vi "Convert Event Level.vi"(4 "Event Level":T2=enum."Info") -> (7 "Enumeration":T1)   [LabVIEW 2020, in "Volatus.lvlib" / "Event Reporter Module.lvclass"]
uses:
  Event Reporter Module.lvclass
  Event Reporter Module.lvclass/Event Reporter Module.ctl
  messages/EventLevel/Enumeration.ctl
  messages/EventLevel/EventLevel.lvlib
  Event Level.ctl
  Volatus.lvlib
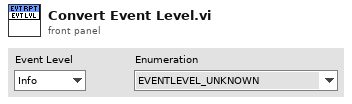
[diagram p1: front panel]
types:
  T1 = typedef "EventLevel.lvlib/Enumeration.ctl" = enum16{"EVENTLEVEL_UNKNOWN", "EVENTLEVEL_DEBUG", "EVENTLEVEL_INFO", "EVENTLEVEL_WARNING", "EVENTLEVEL_ERROR"}
  T2 = typedef "Volatus.lvlib/Event Level.ctl" = enum16{"Debug", "Info", "Warning", "Error"}
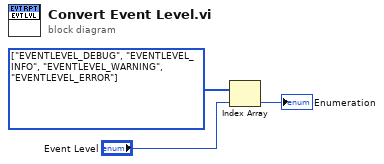
[diagram p0: block diagram]
diagram:
  w3 = T1[] [enum."EVENTLEVEL_DEBUG", enum."EVENTLEVEL_INFO", enum."EVENTLEVEL_WARNING", enum."EVENTLEVEL_ERROR"] items=["EVENTLEVEL_UNKNOWN", "EVENTLEVEL_DEBUG", "EVENTLEVEL_INFO", "EVENTLEVEL_WARNING", "EVENTLEVEL_ERROR"] ("Array")
  n1 = Index Array(array=w3, index="Event Level") -> (element=→"Enumeration":T1)
